vi "Save2.vi"(0 "Save Path":path, 1 "Main folder":string, 2 "DUT":string, 3 "Pass/fail":string, 5 "error in (no error)":errorcluster, 9 "Config":string) -> (14 "Fileout":path, 19 "error out":errorcluster)   [LabVIEW 2024, in "Test_2.lvlib"]
uses:
  Test_2.lvlib
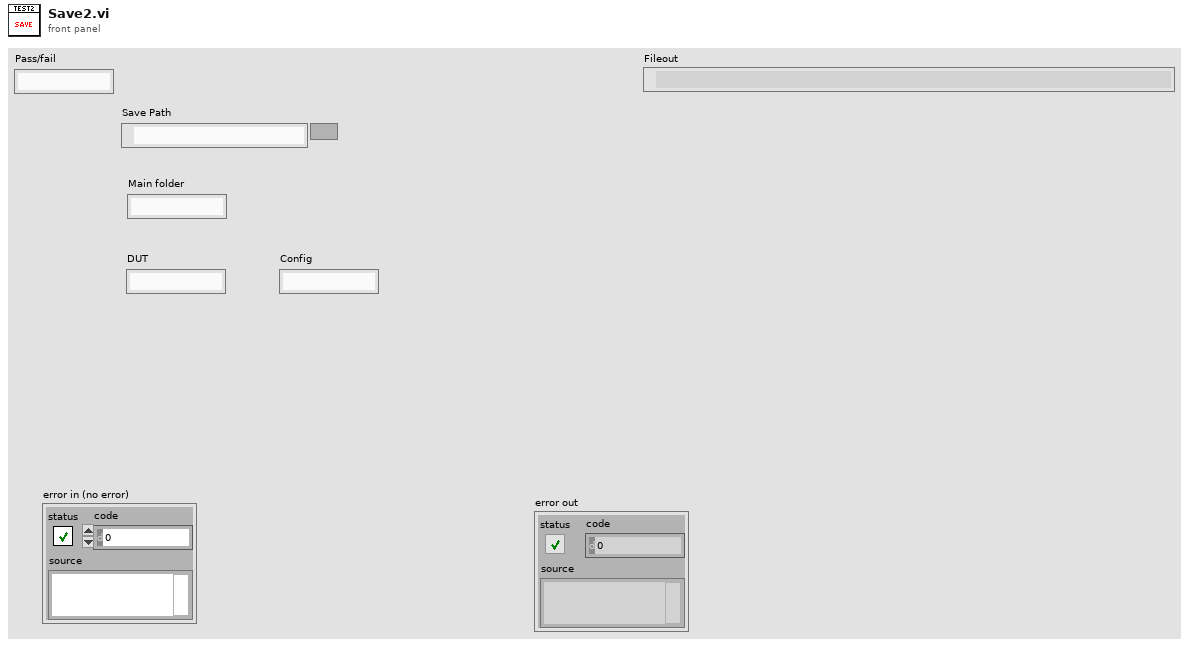
[diagram p1: front panel]
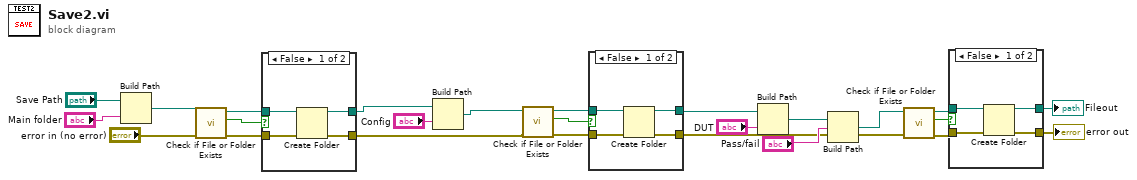
[diagram p0: block diagram]
diagram:
  n1 = Build Path(base path="Save Path", name or relative path="Main folder") -> (appended path=w23:path)
  n2 = call <vilib>:"Check if File or Folder Exists.vi"("error in (no error)"="error in (no error)", "path"=w23) -> ("error out"=w20:errorcluster, "file or folder exists?"=w21:bool, "dup path"=w19:path)  [unwired: 7 in]
  n3 = case shown="False" w21 {
    tunnel: w20 -> [w29 w30]
    tunnel: w19 -> [w28 w31]
    tunnel: [w27 w30] -> w7
    tunnel: [w26 w31] -> w3
    frame False {
      n4 = Create Folder(path (use dialog)=w28, error in=w29) -> (created path=w26:path, error out=w27:errorcluster)  [unwired: 1 in, 1 out]
    }
    frame True {
    }
  }
  n5 = Build Path(base path=w3, name or relative path="Config") -> (appended path=w2:path)
  n6 = call <vilib>:"Check if File or Folder Exists.vi"("error in (no error)"=w7, "path"=w2) -> ("error out"=w6:errorcluster, "file or folder exists?"=w8:bool, "dup path"=w9:path)  [unwired: 7 in]
  n7 = case shown="False" w8 {
    tunnel: w6 -> [w35 w36]
    tunnel: w9 -> [w34 w37]
    tunnel: [w33 w36] -> w5
    tunnel: [w32 w37] -> w4
    frame False {
      n8 = Create Folder(path (use dialog)=w34, error in=w35) -> (created path=w32:path, error out=w33:errorcluster)  [unwired: 1 in, 1 out]
    }
    frame True {
    }
  }
  n9 = Build Path(base path=w4, name or relative path="DUT") -> (appended path=w17:path)
  n10 = Build Path(base path=w17, name or relative path="Pass/fail") -> (appended path=w15:path)
  n11 = call <vilib>:"Check if File or Folder Exists.vi"("error in (no error)"=w5, "path"=w15) -> ("error out"=w13:errorcluster, "file or folder exists?"=w14:bool, "dup path"=w12:path)  [unwired: 7 in]
  n12 = case shown="False" w14 {
    tunnel: w13 -> [w41 w42]
    tunnel: w12 -> [w40 w43]
    tunnel: [w39 w42] -> w10
    tunnel: [w38 w43] -> w11
    frame False {
      n13 = Create Folder(path (use dialog)=w40, error in=w41) -> (created path=w38:path, error out=w39:errorcluster)  [unwired: 1 in, 1 out]
    }
    frame True {
    }
  }
  "Fileout" <- w11
  "error out" <- w10
